vi "Disabled.vi"(7 "Robot Mode":T2, 10 "Match Info":T1={"Autonomous Elapsed Seconds"=0.0, "TeleOp Elapsed Seconds"=0.0, "Disabled Elapsed Seconds"=0.0, "Visited Autonomous"=FALSE, "Visited TeleOp"=FALSE, "Visited Disabled"=FALSE, "Autonomous Settings"={"Autonomous Style"=enum."Independent", "VI Refnum"=refnum}}, 11 "Call Context":T3) -> ()   [LabVIEW 2011]
doc: "This VI is called each time a disabled packet is received from the DS. It is often used to prepare for the next robot mode, to calibrate sensors, etc."
uses:
  <vilib>/Rock Robotics/WPI/DriverStation/WPI_DriverStationDerivedRobotMode.ctl
  <vilib>/Rock Robotics/WPI/DriverStation/WPI_DriverStationRobotMode.ctl
  <vilib>/Rock Robotics/WPI/DriverStation/WPI_DriverStationMatch Info.ctl
  <vilib>/Rock Robotics/WPI/DriverStation/DriverStationLCD/WPI_DriverStationLCDLCDLine.ctl
  Robot Global Data.vi
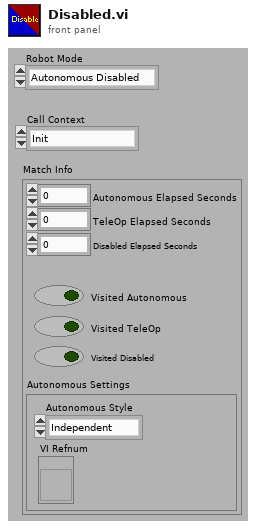
[diagram p1: front panel]
types:
  T1 = typedef "WPI_DriverStationMatch Info.ctl" = cluster{"Autonomous Elapsed Seconds":dbl, "TeleOp Elapsed Seconds":dbl, "Disabled Elapsed Seconds":dbl, "Visited Autonomous":bool, "Visited TeleOp":bool, "Visited Disabled":bool, "Autonomous Settings":cluster{"Autonomous Style":enum16{"Iterative", "Independent"}, "VI Refnum":refnum<vi>}}
  T2 = typedef "WPI_DriverStationRobotMode.ctl" = enum16{"Autonomous Disabled", "Autonomous Enabled", "Teleop Disabled", "Teleop Enabled", "Timeout", "Finish"}
  T3 = typedef "WPI_DriverStationDerivedRobotMode.ctl" = enum16{"Init", "Execute", "Stop"}
  T4 = typedef "WPI_DriverStationLCDLCDLine.ctl" = enum16{"Main - Line 1", "User - Line 2", "User - Line 3", "User - Line 4", "User - Line 5", "User - Line 6"}
  T5 = typedef "WPI_MotorControlDeviceRef.ctl" = cluster{"DeviceStatus":errorcluster, "Type":enum16{"PWM", "CAN"}, "PWM":cluster{"Digital Module":T6, "PWM Channel":T7, "DeadBand":T8}, "CAN":cluster{"Device Number":u8, "Control Mode":T9, "Semaphore":T10, "Max Vout":dbl}, "Invert":bool, "TransformRef":T11, "InvTransformRef":T11}
  T6 = typedef "FPGA_TypedefDigitalModule.ctl" = enum16{"Digital Module 1", "Digital Module 2"}
  T7 = typedef "FPGA_DIOPWMChannel.ctl" = enum8{"PWM 1", "PWM 2", "PWM 3", "PWM 4", "PWM 5", "PWM 6", "PWM 7", "PWM 8", "PWM 9", "PWM 10", "Invalid"}
  T8 = typedef "WPI_PWMDeadband.ctl" = cluster{"Name":string, "maxPositivePwm":i32, "minPositivePwm":i32, "centerPwm":i32, "maxNegativePwm":i32, "minNegativePwm":i32, "angularRange":u16}
  T9 = typedef "WPI_CANJaguar_ControlMode.ctl" = enum8{"Percent VBus", "Current", "Speed", "Position", "Voltage"}
  T10 = typedef "Semaphore RefNum" = refnum<k1>
  T11 = typedef "WPI_PWMTransform_ConPane.ctl" = refnum<vi>
  T12 = typedef "WPI_JoystickDevRef.ctl" = cluster{"Device":T13}
  T13 = typedef "WPI_JoystickDeviceEnum.ctl" = enum16{"USB 1", "USB 2", "USB 3", "USB 4", "Kinect 1", "Kinect 2"}
  T14 = typedef "WPI_JoystickButtonState.ctl" = cluster{"Button 1":bool, "Button 2":bool, "Button 3":bool, "Button 4":bool, "Button 5":bool, "Button 6":bool, "Button 7":bool, "Button 8":bool, "Button 9":bool, "Button 10":bool, "Button 11":bool, "Button 12":bool}
  T15 = typedef "WPI_ServoDeviceRef.ctl" = cluster{"DeviceStatus":errorcluster, "Digital Module":T6, "PWM Channel":T7, "DeadBand":T8}
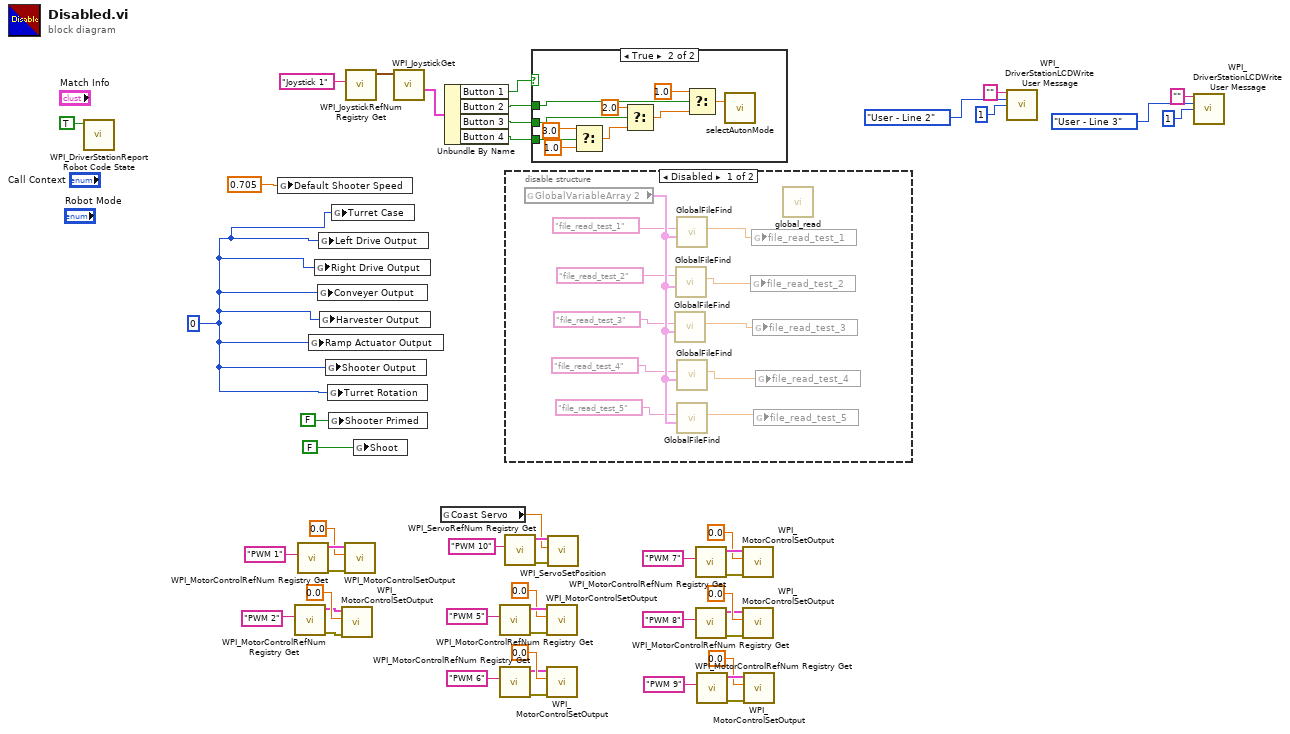
[diagram p0: block diagram]
diagram:
  w19 = 0
  n1 = call <vilib>:"WPI_DriverStationReport Robot Code State.vi"("Disabled"=TRUE ("Autonomous")) -> ()  [unwired: 10 in, 1 out]
  n2 = global write "Robot Global Data.vi" "Default Shooter Speed"(0.705 ("Balls in Robot")) -> ()
  n3 = call <vilib>:"WPI_MotorControlRefNum Registry Get.vi"("refnum name"="PWM 2") -> ("error out"=w43:errorcluster, "MotorControlDevRef"=w42:T5)  [unwired: 9 in]
  n4 = call <vilib>:"WPI_MotorControlRefNum Registry Get.vi"("refnum name"="PWM 1") -> ("error out"=w48:errorcluster, "MotorControlDevRef"=w49:T5)  [unwired: 9 in]
  n5 = global write "Robot Global Data.vi" "Ramp Actuator Output"(w19) -> ()
  n6 = global write "Robot Global Data.vi" "Right Drive Output"(w19) -> ()
  n7 = global write "Robot Global Data.vi" "Conveyer Output"(w19) -> ()
  n8 = global write "Robot Global Data.vi" "Left Drive Output"(w19) -> ()
  n9 = global write "Robot Global Data.vi" "Harvester Output"(w19) -> ()
  n10 = global write "Robot Global Data.vi" "Shooter Output"(w19) -> ()
  n11 = global write "Robot Global Data.vi" "Turret Rotation"(w19) -> ()
  n12 = global write "Robot Global Data.vi" "Shooter Primed"(FALSE ("Shooter Primed")) -> ()
  n13 = global write "Robot Global Data.vi" "Turret Case"(w19) -> ()
  n14 = call <vilib>:"WPI_MotorControlSetOutput.vi"("error in (no error)"=w43, "Output"=0.0, "MotorControlDevRef"=w42) -> ()  [unwired: 7 in, 2 out]
  n15 = call <vilib>:"WPI_MotorControlSetOutput.vi"("error in (no error)"=w48, "Output"=0.0, "MotorControlDevRef"=w49) -> ()  [unwired: 7 in, 2 out]
  n16 = call <vilib>:"WPI_JoystickRefNum Registry Get.vi"("refnum name"="Joystick 1") -> ("JoystickDevRef"=w17:T12)  [unwired: 9 in, 1 out]
  n17 = global write "Robot Global Data.vi" "Shoot"(FALSE ("Shooter Primed")) -> ()
  n18 = call <vilib>:"WPI_JoystickGet.vi"("JoystickDevRef"=w17) -> ("Buttons"=w16:T14)  [unwired: 4 in, 2 out]
  n19 = global read "Robot Global Data.vi" "Coast Servo"() -> (w2:dbl)
  n20 = Unbundle By Name(w16) -> ("Button 1"=w15:bool, "Button 2"=w14:bool, "Button 3"=w13:bool, "Button 4"=w12:bool)
  n21 = call <vilib>:"WPI_MotorControlRefNum Registry Get.vi"("refnum name"="PWM 5") -> ("error out"=w40:errorcluster, "MotorControlDevRef"=w41:T5)  [unwired: 9 in]
  n22 = call <vilib>:"WPI_MotorControlRefNum Registry Get.vi"("refnum name"="PWM 6") -> ("error out"=w35:errorcluster, "MotorControlDevRef"=w34:T5)  [unwired: 9 in]
  n23 = call <vilib>:"WPI_ServoRefNum Registry Get.vi"("refnum name"="PWM 10") -> ("error out"=w4:errorcluster, "ServoDeviceRef"=w3:T15)  [unwired: 9 in]
  n24 = disable-structure shown="Disabled" {
    frame Disabled {
      n25 = global read "Robot Global Data.vi" "GlobalVariableArray 2"() -> (w61:cluster{"name":string, "va;":dbl}[])
      n26 = call "GlobalFileFind.vi"("GlobalVariableArray 2"=w61, "VariableNameLookup"="file_read_test_3") -> ("VariableValueOut"=w52:dbl)  [unwired: 9 in]
      n27 = call "GlobalFileFind.vi"("GlobalVariableArray 2"=w61, "VariableNameLookup"="file_read_test_2") -> ("VariableValueOut"=w51:dbl)  [unwired: 9 in]
      n28 = call "GlobalFileFind.vi"("GlobalVariableArray 2"=w61, "VariableNameLookup"="file_read_test_1") -> ("VariableValueOut"=w55:dbl)  [unwired: 9 in]
      n29 = call "GlobalFileFind.vi"("GlobalVariableArray 2"=w61, "VariableNameLookup"="file_read_test_4") -> ("VariableValueOut"=w53:dbl)  [unwired: 9 in]
      n30 = call "GlobalFileFind.vi"("GlobalVariableArray 2"=w61, "VariableNameLookup"="file_read_test_5") -> ("VariableValueOut"=w54:dbl)  [unwired: 9 in]
      n31 = global write "Robot Global Data.vi" "file_read_test_2"(w51) -> ()
      n32 = global write "Robot Global Data.vi" "file_read_test_1"(w55) -> ()
      n33 = global write "Robot Global Data.vi" "file_read_test_3"(w52) -> ()
      n34 = global write "Robot Global Data.vi" "file_read_test_5"(w54) -> ()
      n35 = global write "Robot Global Data.vi" "file_read_test_4"(w53) -> ()
      n36 = call "global_read.vi"() -> ()  [unwired: 12 in]
    }
    frame Enabled {
    }
  }
  n37 = case shown="True" w15 {
    tunnel: w14 -> [_ w68]
    tunnel: w13 -> [_ w66]
    tunnel: w12 -> [_ w71]
    frame False {
    }
    frame True {
      n38 = Select(t=3.0, s=w71, f=1.0) -> (s? t:f=w64:dbl)
      n39 = Select(t=2.0, s=w66, f=w64) -> (s? t:f=w63:dbl)
      n40 = Select(t=1.0, s=w68, f=w63) -> (s? t:f=w62:dbl)
      n41 = call "selectAutonMode.vi"("Auton File"=w62) -> ()  [unwired: 2 in]
    }
  }
  n42 = call <vilib>:"WPI_MotorControlSetOutput.vi"("error in (no error)"=w40, "Output"=0.0, "MotorControlDevRef"=w41) -> ()  [unwired: 7 in, 2 out]
  n43 = call <vilib>:"WPI_MotorControlSetOutput.vi"("error in (no error)"=w35, "Output"=0.0, "MotorControlDevRef"=w34) -> ()  [unwired: 7 in, 2 out]
  n44 = call <vilib>:"WPI_ServoSetPosition.vi"("error in (no error)"=w4, "Position"=w2, "ServoDeviceRef"=w3) -> ()  [unwired: 7 in, 2 out]
  n45 = call <vilib>:"WPI_MotorControlRefNum Registry Get.vi"("refnum name"="PWM 7") -> ("error out"=w32:errorcluster, "MotorControlDevRef"=w33:T5)  [unwired: 9 in]
  n46 = call <vilib>:"WPI_MotorControlRefNum Registry Get.vi"("refnum name"="PWM 8") -> ("error out"=w27:errorcluster, "MotorControlDevRef"=w26:T5)  [unwired: 9 in]
  n47 = call <vilib>:"WPI_MotorControlRefNum Registry Get.vi"("refnum name"="PWM 9") -> ("error out"=w24:errorcluster, "MotorControlDevRef"=w25:T5)  [unwired: 9 in]
  n48 = call <vilib>:"WPI_MotorControlSetOutput.vi"("error in (no error)"=w32, "Output"=0.0, "MotorControlDevRef"=w33) -> ()  [unwired: 7 in, 2 out]
  n49 = call <vilib>:"WPI_MotorControlSetOutput.vi"("error in (no error)"=w27, "Output"=0.0, "MotorControlDevRef"=w26) -> ()  [unwired: 7 in, 2 out]
  n50 = call <vilib>:"WPI_MotorControlSetOutput.vi"("error in (no error)"=w24, "Output"=0.0, "MotorControlDevRef"=w25) -> ()  [unwired: 7 in, 2 out]
  n51 = call <vilib>:"WPI_DriverStationLCDWrite User Message.vi"("line text"="", "line"=WPI_DriverStationLCDLCDLine."User - Line 2", "starting column"=i8 1) -> ()  [unwired: 2 in, 11 out]
  n52 = call <vilib>:"WPI_DriverStationLCDWrite User Message.vi"("line text"="", "line"=WPI_DriverStationLCDLCDLine."User - Line 3", "starting column"=i8 1) -> ()  [unwired: 2 in, 11 out]
